vi "Clear Error.vi"(7 "code":i32, 8 "error in (no error)":errorcluster, 11 "prev clear":bool) -> (0 "error out":errorcluster, 3 "clear":bool)   [LabVIEW 2014, in "lvprj2html.lvlib"]
uses:
  lvprj2html.lvlib
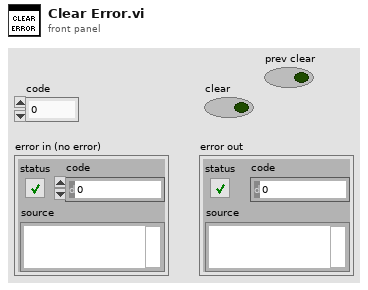
[diagram p1: front panel]
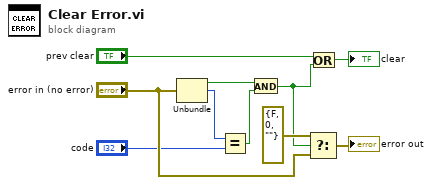
[diagram p0: block diagram]
diagram:
  n1 = Unbundle("error in (no error)") -> ("status"=w4:bool, "code"=w5:i32)  [unwired: 1 out]
  n2 = Equal?(x=w5, y="code") -> (x = y?=w8:bool)
  n3 = And(x=w4, y=w8) -> (x .and. y?=w3:bool)
  n4 = Select(t=errorcluster {"status"=FALSE, "code"=0, "source"=""}, s=w3, f="error in (no error)") -> (s? t:f=→"error out":errorcluster)
  n5 = Or(x="prev clear", y=w3) -> (x .or. y?=→"clear":bool)
